vi "Display Picture.vi"(4 "Comment":string, 6 "Fetch":bool, 8 "depth":i32=24, 9 "rect":T1={"left"=0, "top"=0, "right"=640, "bottom"=400}, 10 "picture":picture, 11 "error in":errorcluster) -> (3 "error out":errorcluster)   [LabVIEW 2013]
uses:
  ROS/Code/SubVIs/BaxterCamera.ctl
panel:
  in  "node":string
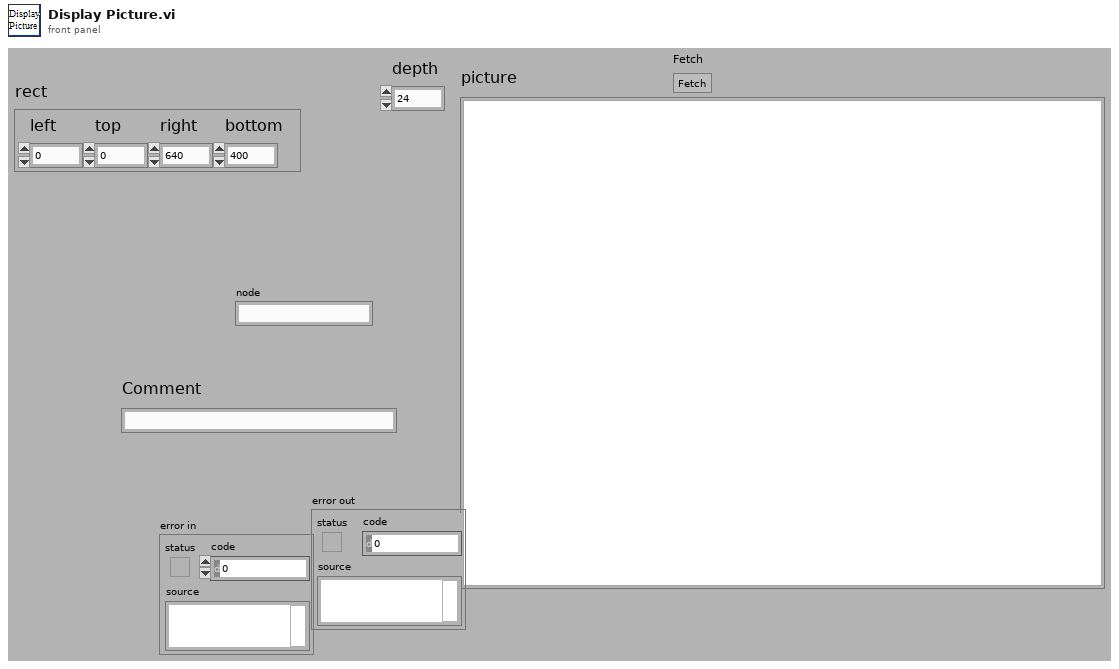
[diagram p1: front panel]
types:
  T1 = cluster{"left":i16, "top":i16, "right":i16, "bottom":i16}
  T2 = cluster{"Height":u32, "Width":u32, "is_bigendian?":u8, "Step":u32, "Data":u8[], "Encoding":string, "Frame ID":string}
  T3 = cluster{"Font Name:":string, "Size":i16, "Strikeout?":bool, "Italic?":bool, "Underline?":bool, "Outline?":bool, "Shadow?":bool, "Bold?":bool}
  T4 = enum16{"User-specified Font", "Application Font", "System Font", "Dialog Font"}
  T5 = typedef "BaxterCamera.ctl" = enum16{"left_hand_camera", "right_hand_camera", "head_camera"}
  T6 = typedef "LVBoundsTypeDef.ctl" = cluster{"Width":u32, "Height":u32}
  T7 = typedef "imagedata.ctl" = cluster{"image type":i32, "image depth":i32, "image":u8[], "mask":u8[], "colors":u32[], "Rectangle":cluster{"left":i16, "top":i16, "right":i16, "bottom":i16}}
  T8 = typedef "_ROSControl.ctl" = cluster{"topic port":u16, "Node":string, "topic":string, "type":string, "node port":u32, "error ":errorcluster, "Direction":T9, "APIs":string[]}
  T9 = typedef "_ROSDirection.ctl" = enum16{"Node", "Publisher", "Subscriber", "Service Client"}
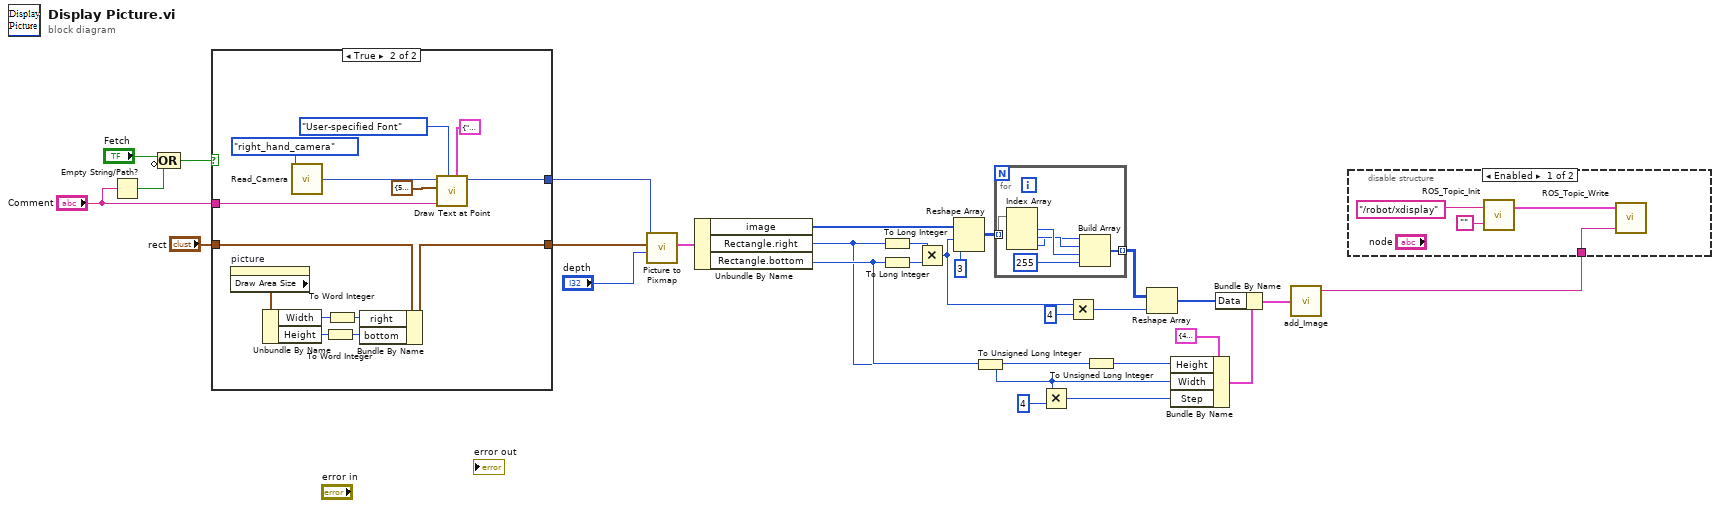
[diagram p0: block diagram]
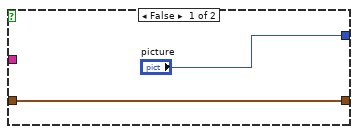
[diagram p2: hidden frame]
diagram:
  n1 = Empty String/Path?(string/path="Comment") -> (empty?=w2:bool)
  n2 = Compound Arithmetic op=OR("Fetch", invert w2) -> (w4:bool)
  n3 = case shown="True" w4 {
    tunnel: ["picture" w36] -> w7
    tunnel: [w30 w42] -> w6
    tunnel: "rect" -> [w30 w43]
    tunnel: "Comment" -> [_ w32]
    frame False {
    }
    frame True {
      n4 = property on="picture" class="Pict"() -> ("Draw Area Size"=w41:T6)  [unwired: 2 in, 2 out]
      n5 = Unbundle By Name(w41) -> ("Width"=w40:u32, "Height"=w39:u32)
      n6 = call "Read_Camera.vi"("Camera"=BaxterCamera."right_hand_camera") -> ("picture"=w44:picture)  [unwired: 2 in, 4 out]
      n7 = To Word Integer(number=w39) -> (16bit integer=w37:i16)
      n8 = To Word Integer(number=w40) -> (16bit integer=w38:i16)
      n9 = Bundle By Name(cluster=w43, "right"=w38, "bottom"=w37) -> (w42:T1)
      n10 = call <vilib>:"Draw Text at Point.vi"("[user-specified font]"=T3 {"Font Name:"="Arial Black", "Size"=80, "Strikeout?"=FALSE, "Italic?"=FALSE, "Underline?"=FALSE, "Outline?"=FALSE, "Shadow?"=FALSE, "Bold?"=TRUE}, "desired font(Application)"=T4."User-specified Font", "text"=w32, "origin"=cluster{"x":i16, "y":i16} {"x"=50, "y"=420}, "picture"=w44) -> ("new picture"=w36:picture)  [unwired: 5 in, 1 out]
    }
  }
  n11 = call <vilib>:"Picture to Pixmap.vi"("depth"="depth", "rect"=w6, "picture"=w7) -> ("image data"=w28:T7)  [unwired: 7 in, 1 out]
  n12 = Unbundle By Name(w28) -> ("image"=w27:u8[], "Rectangle.right"=w10:i16, "Rectangle.bottom"=w13:i16)
  n13 = To Long Integer(number=w10) -> (32bit integer=w24:i32)
  n14 = To Long Integer(number=w13) -> (32bit integer=w23:i32)
  n15 = Multiply(x=w24, y=w23) -> (x*y=w20:i32)
  n16 = Reshape Array(w27, w20, 3 ("dimension size")) -> (w19:u8[][])
  n17 = To Unsigned Long Integer(number=w10) -> (unsigned 32bit integer=w8:u32)
  n18 = for {
    tunnel: w19 -> [w49] mode=indexing
    tunnel: [w50] -> w18 mode=indexing
    n19 = Index Array(array=w49) -> (element #1=w48:u8, element #2=w47:u8, element #3=w46:u8)  [unwired: 3 in]
    n20 = Build Array(w46, w47, w48, u8 255 ("element")) -> (w50:u8[])
  }
  n21 = Multiply(x=w8, y=u32 4) -> (x*y=w11:u32)
  n22 = Multiply(x=w20, y=4) -> (x*y=w25:i32)
  n23 = To Unsigned Long Integer(number=w13) -> (unsigned 32bit integer=w12:u32)
  n24 = Reshape Array(w18, w25) -> (w22:u8[])
  n25 = Bundle By Name(cluster=T2 {"Height"=400, "Width"=640, "is_bigendian?"=0, "Step"=2560, "Data"=[], "Encoding"="bgra8", "Frame ID"="NIST"} ("ROS Image"), "Height"=w12, "Width"=w8, "Step"=w11) -> (w14:T2)
  n26 = Bundle By Name(cluster=w14, "Data"=w22) -> (w29:T2)
  n27 = call "add_Image.vi"("ROS Image"=w29) -> ("msg out"=w17:string)  [unwired: 4 in]
  n28 = disable-structure shown="Enabled" {
    disable-tunnel: w17 -> [w55 _]
    frame Enabled {
      n29 = call "ROS_Topic_Init.vi"("node"="", "topic"="/robot/xdisplay") -> ("ROS out"=w53:T8)  [unwired: 1 in]
      n30 = call "ROS_Topic_Write.vi"("Msg in"=w55, "ROS in"=w53) -> ()  [unwired: 2 in, 1 out]
    }
    frame Disabled {
    }
  }
